vi "Visible Label.vi"(8 "error in (no error)":errorcluster, 10 "label":enum8{"hide", "show"}(ring), 11 "GObject in":refnum<vi>) -> (0 "error out":errorcluster, 1 "was label visible?":enum8{"hide", "show"}(ring), 2 "has label?":bool, 3 "GObject out":refnum<vi>)   [LabVIEW 2019, in "Builtins.lvlib"]
doc: "Shows or hides the GObject label if exists.\n\nCreated by: Ryan Pacini"
uses:
  Builtins.lvlib
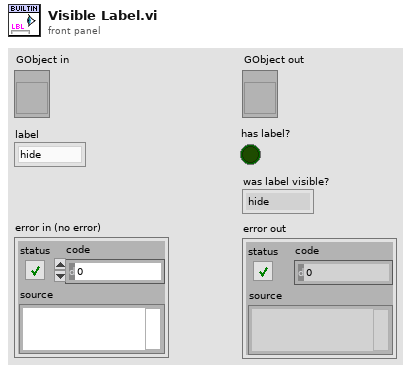
[diagram p1: front panel]
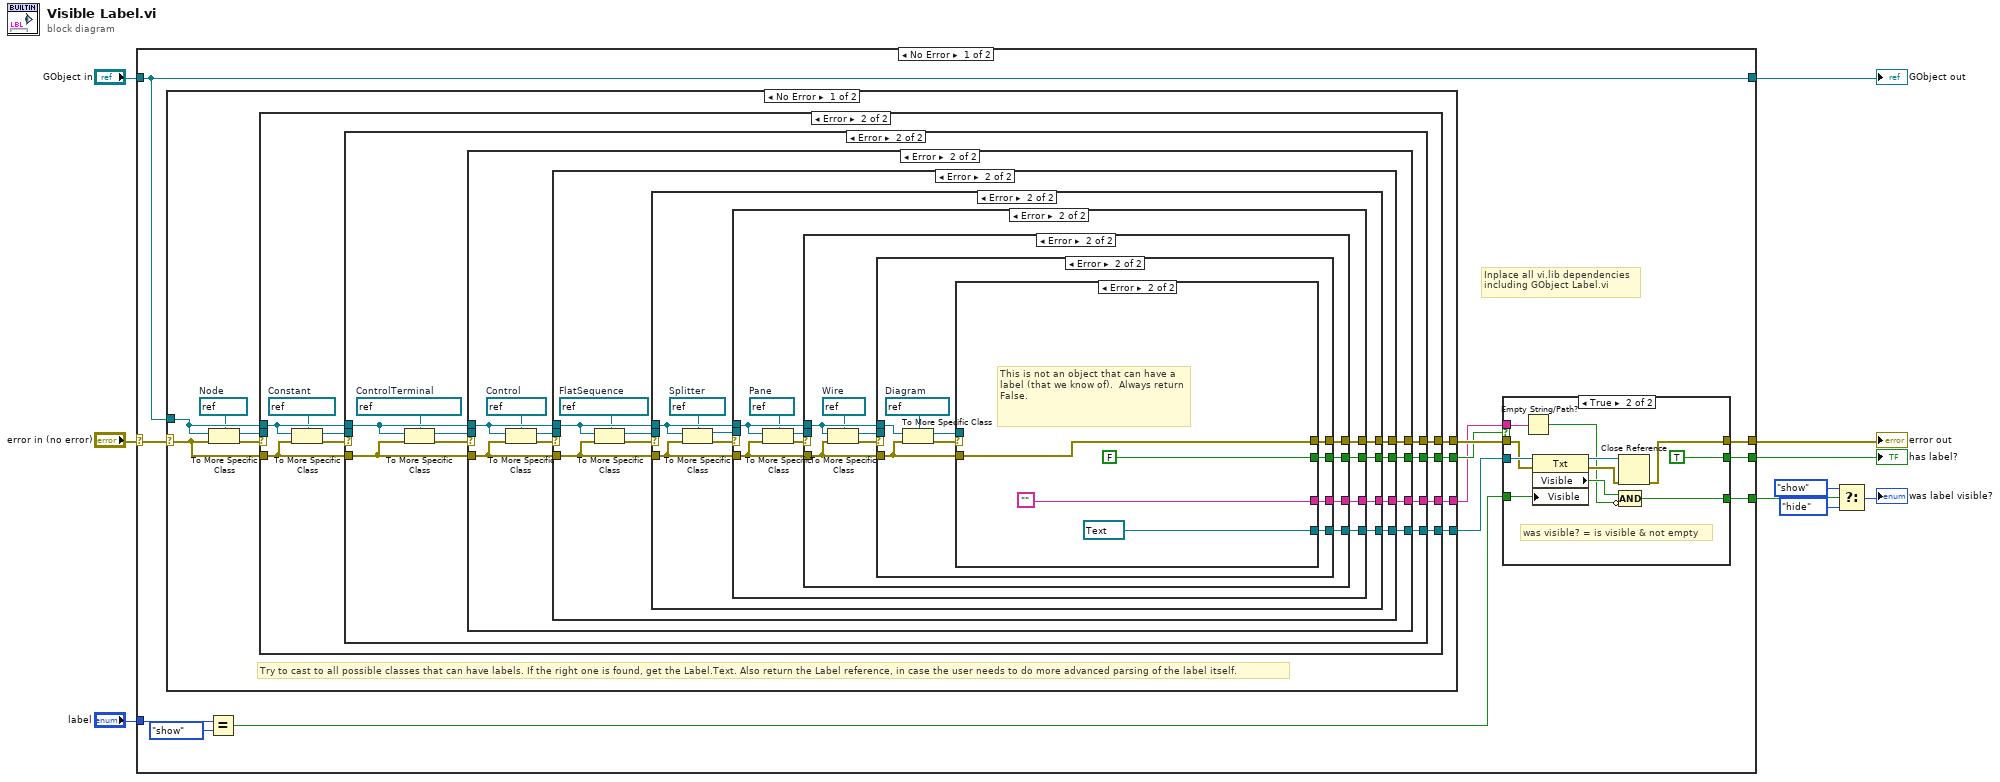
[diagram p0: block diagram]
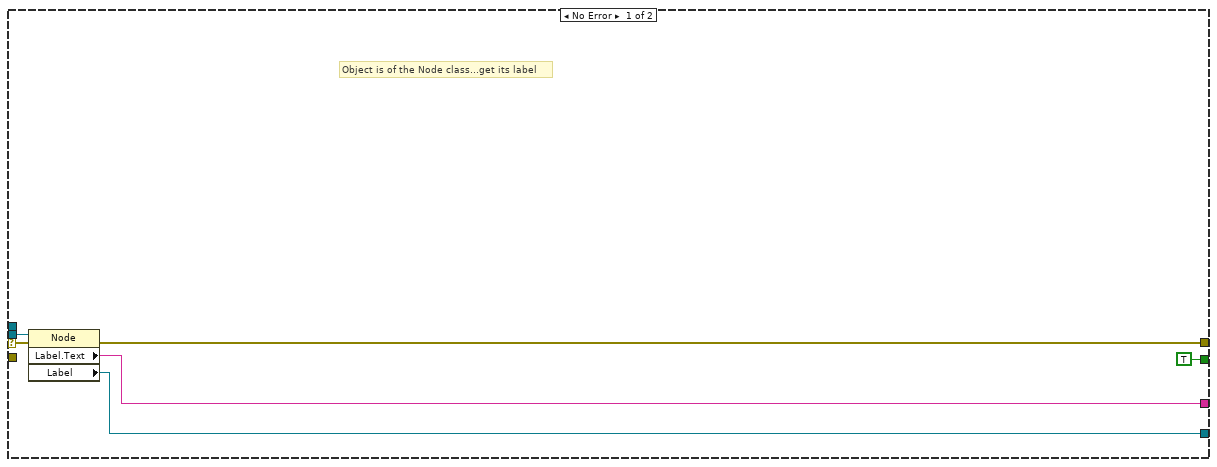
[diagram p2: hidden frame]
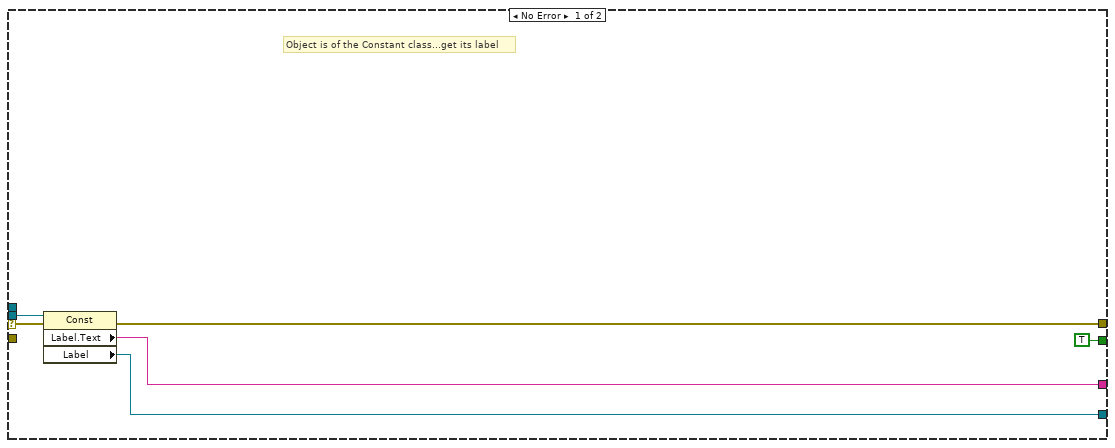
[diagram p3: hidden frame]
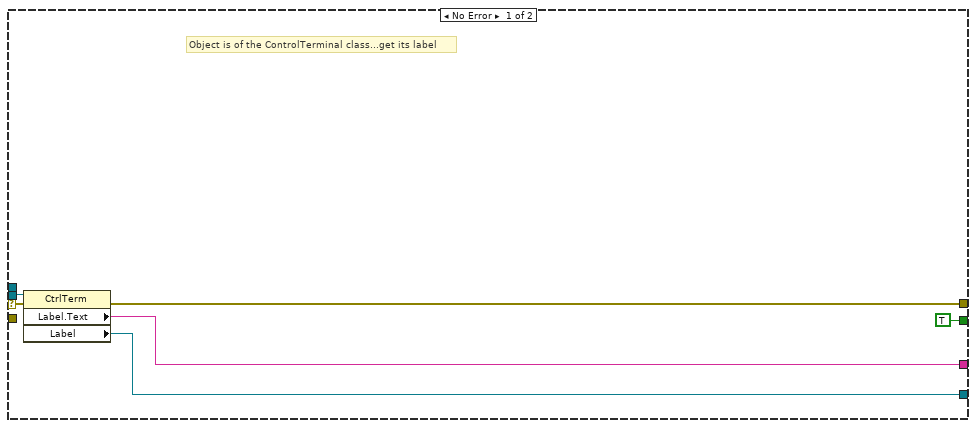
[diagram p4: hidden frame]
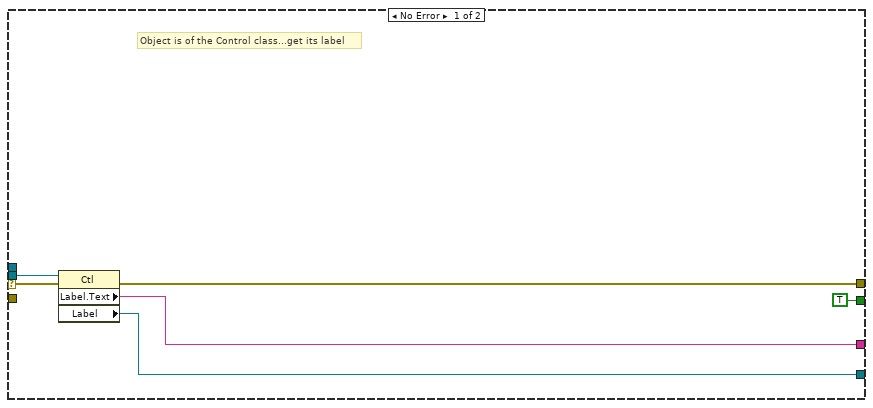
[diagram p5: hidden frame]
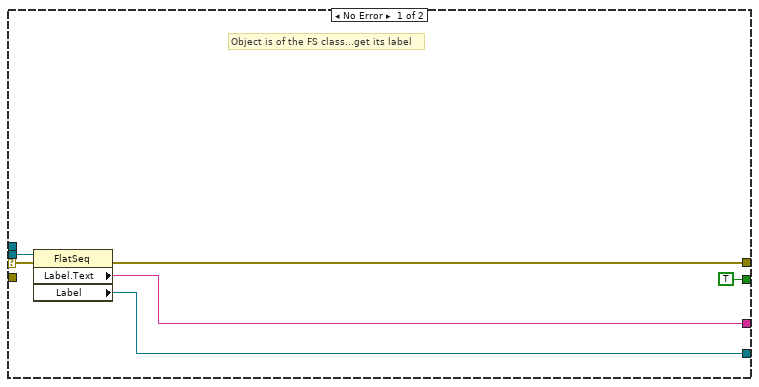
[diagram p6: hidden frame]
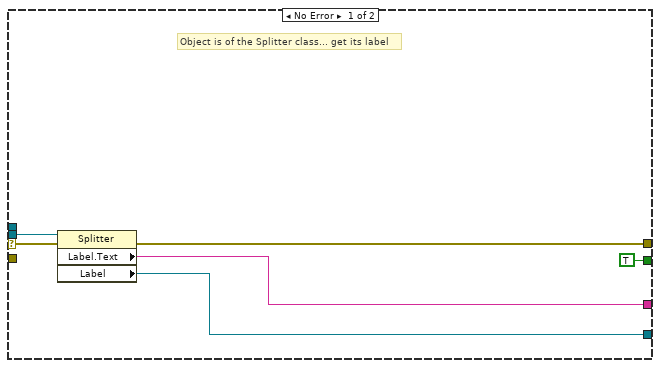
[diagram p7: hidden frame]
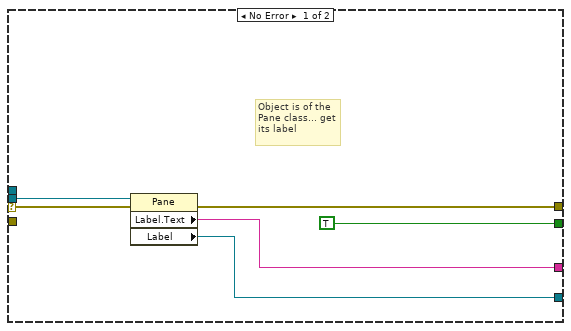
[diagram p8: hidden frame]
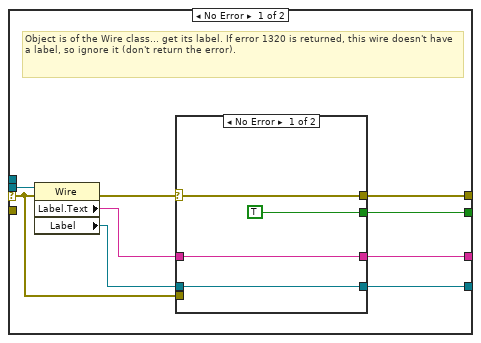
[diagram p9: hidden frame]
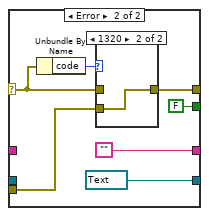
[diagram p10: hidden frame]
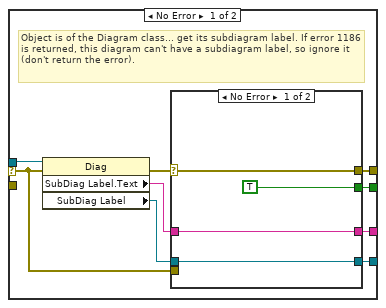
[diagram p12: hidden frame]
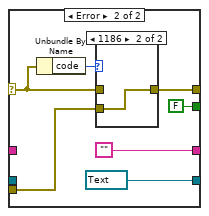
[diagram p13: hidden frame]
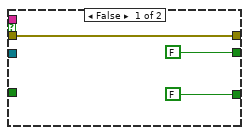
[diagram p16: hidden frame]
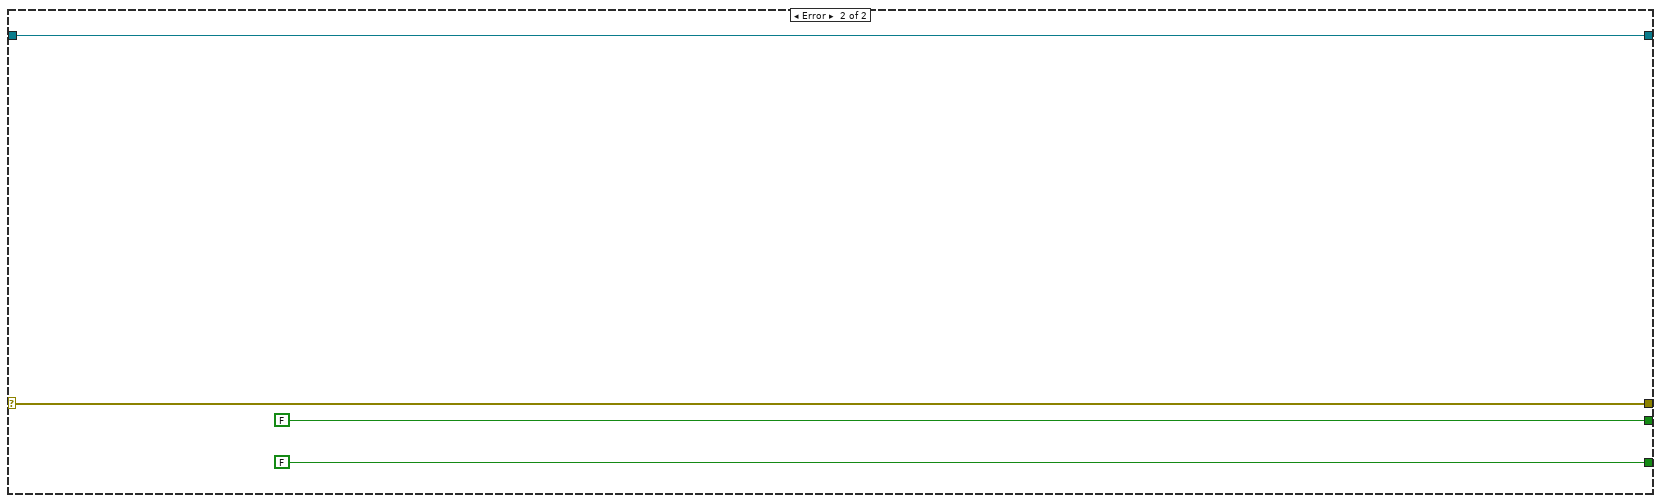
[diagram p17: hidden frame]
diagram:
  n1 = case shown="No Error" "error in (no error)" {
    selector: "error in (no error)" -> [w22 w211]
    tunnel: "label" -> [w14 _]
    tunnel: [w19 FALSE ("Visible")] -> w5
    tunnel: [w18 w211] -> w4
    tunnel: "GObject in" -> [w16 w212]
    tunnel: [w16 w212] -> w2
    tunnel: [w15 FALSE] -> w1
    frame No Error {
      # "Inplace all vi.lib dependencies\nincluding GObject Label.vi"
      n2 = case shown="No Error" w22 {
        selector: w22 -> [w27 w194]
        tunnel: w16 -> [w26 _]
        tunnel: [w31 w194] -> w20
        tunnel: [w30 _] -> w17
        tunnel: [w25 _] -> w11
        tunnel: [w24 _] -> w21
        frame No Error {
          w23 = refnum<vi> refnum  # Node
          # "Try to cast to all possible classes that can have labels. If the right one is found, get the Label.Text. Also return the Label reference, in case the user needs to do more advanced parsing of the label itself."
          n3 = To More Specific Class(target class=w23, reference=w26, error in=w27) -> (specific class reference=w28:refnum<vi>, error out=w29:errorcluster)
          n4 = case shown="Error" w29 {
            selector: w29 -> [w37 _]
            tunnel: w26 -> [_ w44]
            tunnel: w28 -> [w36 _]
            tunnel: w27 -> [_ w43]
            tunnel: [TRUE w42] -> w30
            tunnel: [w35 w41] -> w31
            tunnel: [w33 w40] -> w25
            tunnel: [w32 w39] -> w24
            frame No Error {
              # "Object is of the Node class...get its label"
              n5 = property class="Node"(reference=w36, error in=w37) -> (error out=w35:errorcluster, "Label.Text"=w33:string, "Label"=w32:refnum<vi>)  [unwired: 1 out]
            }
            frame Error {
              w38 = refnum<vi> refnum  # Constant
              n6 = To More Specific Class(target class=w38, reference=w44, error in=w43) -> (specific class reference=w45:refnum<vi>, error out=w46:errorcluster)
              n7 = case shown="Error" w46 {
                selector: w46 -> [w52 _]
                tunnel: w45 -> [w51 _]
                tunnel: w44 -> [_ w59]
                tunnel: w43 -> [_ w58]
                tunnel: [TRUE w56] -> w42
                tunnel: [w50 w57] -> w41
                tunnel: [w48 w55] -> w40
                tunnel: [w47 w54] -> w39
                frame No Error {
                  # "Object is of the Constant class...get its label"
                  n8 = property class="Const"(reference=w51, error in=w52) -> (error out=w50:errorcluster, "Label.Text"=w48:string, "Label"=w47:refnum<vi>)  [unwired: 1 out]
                }
                frame Error {
                  w53 = refnum<vi> refnum  # ControlTerminal
                  n9 = To More Specific Class(target class=w53, reference=w59, error in=w58) -> (specific class reference=w60:refnum<vi>, error out=w61:errorcluster)
                  n10 = case shown="Error" w61 {
                    selector: w61 -> [w67 _]
                    tunnel: w60 -> [w66 _]
                    tunnel: w59 -> [_ w74]
                    tunnel: w58 -> [_ w73]
                    tunnel: [w65 w72] -> w57
                    tunnel: [TRUE w71] -> w56
                    tunnel: [w64 w70] -> w55
                    tunnel: [w62 w69] -> w54
                    frame No Error {
                      # "Object is of the ControlTerminal class...get its label"
                      n11 = property class="CtrlTerm"(reference=w66, error in=w67) -> (error out=w65:errorcluster, "Label.Text"=w64:string, "Label"=w62:refnum<vi>)  [unwired: 1 out]
                    }
                    frame Error {
                      w68 = refnum<vi> refnum  # Control
                      n12 = To More Specific Class(target class=w68, reference=w74, error in=w73) -> (specific class reference=w75:refnum<vi>, error out=w76:errorcluster)
                      n13 = case shown="Error" w76 {
                        selector: w76 -> [w82 _]
                        tunnel: w75 -> [w81 _]
                        tunnel: w74 -> [_ w86]
                        tunnel: w73 -> [_ w89]
                        tunnel: [w80 w87] -> w72
                        tunnel: [TRUE w88] -> w71
                        tunnel: [w79 w85] -> w70
                        tunnel: [w77 w84] -> w69
                        frame No Error {
                          # "Object is of the Control class...get its label"
                          n14 = property class="Ctl"(reference=w81, error in=w82) -> (error out=w80:errorcluster, "Label.Text"=w79:string, "Label"=w77:refnum<vi>)  [unwired: 1 out]
                        }
                        frame Error {
                          w83 = refnum<vi> refnum  # FlatSequence
                          n15 = To More Specific Class(target class=w83, reference=w86, error in=w89) -> (specific class reference=w90:refnum<vi>, error out=w91:errorcluster)
                          n16 = case shown="Error" w91 {
                            selector: w91 -> [w97 _]
                            tunnel: w90 -> [w96 _]
                            tunnel: w89 -> [_ w104]
                            tunnel: [TRUE w101] -> w88
                            tunnel: [w95 w102] -> w87
                            tunnel: w86 -> [_ w105]
                            tunnel: [w94 w100] -> w85
                            tunnel: [w92 w99] -> w84
                            frame No Error {
                              # "Object is of the FS class...get its label"
                              n17 = property class="FlatSeq"(reference=w96, error in=w97) -> (error out=w95:errorcluster, "Label.Text"=w94:string, "Label"=w92:refnum<vi>)  [unwired: 1 out]
                            }
                            frame Error {
                              w98 = refnum<vi> refnum  # Splitter
                              n18 = To More Specific Class(target class=w98, reference=w105, error in=w104) -> (specific class reference=w103:refnum<vi>, error out=w106:errorcluster)
                              n19 = case shown="Error" w106 {
                                selector: w106 -> [w110 _]
                                tunnel: w105 -> [_ w115]
                                tunnel: w104 -> [_ w120]
                                tunnel: w103 -> [w112 _]
                                tunnel: [w111 w119] -> w102
                                tunnel: [TRUE w118] -> w101
                                tunnel: [w109 w116] -> w100
                                tunnel: [w107 w114] -> w99
                                frame No Error {
                                # "Object is of the Splitter class... get its label"
                                n20 = property class="Splitter"(reference=w112, error in=w110) -> (error out=w111:errorcluster, "Label.Text"=w109:string, "Label"=w107:refnum<vi>)  [unwired: 1 out]
                                }
                                frame Error {
                                w113 = refnum<vi> refnum  # Pane
                                n21 = To More Specific Class(target class=w113, reference=w115, error in=w120) -> (specific class reference=w117:refnum<vi>, error out=w121:errorcluster)
                                n22 = case shown="Error" w121 {
                                selector: w121 -> [w127 _]
                                tunnel: w120 -> [_ w132]
                                tunnel: [w125 w131] -> w119
                                tunnel: [TRUE w136] -> w118
                                tunnel: w117 -> [w126 _]
                                tunnel: [w124 w135] -> w116
                                tunnel: w115 -> [_ w130]
                                tunnel: [w122 w129] -> w114
                                frame No Error {
                                # "Object is of the Pane class... get its label"
                                n23 = property class="Pane"(reference=w126, error in=w127) -> (error out=w125:errorcluster, "Label.Text"=w124:string, "Label"=w122:refnum<vi>)  [unwired: 1 out]
                                }
                                frame Error {
                                w128 = refnum<vi> refnum  # Wire
                                n24 = To More Specific Class(target class=w128, reference=w130, error in=w132) -> (specific class reference=w133:refnum<vi>, error out=w134:errorcluster)
                                n25 = case shown="Error" w134 {
                                selector: w134 -> [w141 _]
                                tunnel: [w139 w167] -> w136
                                tunnel: [w138 w166] -> w135
                                tunnel: w133 -> [w145 _]
                                tunnel: w132 -> [_ w162]
                                tunnel: [w140 w161] -> w131
                                tunnel: w130 -> [_ w165]
                                tunnel: [w137 w160] -> w129
                                frame No Error {
                                # "Object is of the Wire class... get its label. If error 1320 is returned, this wire doesn't have a label, so ignore it (don't return the error)."
                                n26 = property class="Wire"(reference=w145, error in=w141) -> (error out=w144:errorcluster, "Label.Text"=w143:string, "Label"=w142:refnum<vi>)  [unwired: 1 out]
                                n27 = case shown="No Error" w144 {
                                selector: w144 -> [w149 w155]
                                tunnel: [w149 w152] -> w140
                                tunnel: w143 -> [w148 _]
                                tunnel: [w148 ""] -> w138
                                tunnel: w142 -> [w146 _]
                                tunnel: [w146 refnum<vi> refnum ("SubDiag Label")] -> w137
                                tunnel: [TRUE FALSE] -> w139
                                tunnel: w141 -> [_ w150]
                                frame No Error {
                                }
                                frame Error {
                                n28 = Unbundle By Name(w155) -> ("code"=w156:i32)
                                n29 = case shown="1320" w156 {
                                tunnel: w155 -> [w157 _]
                                tunnel: [w157 w158] -> w152
                                tunnel: w150 -> [_ w158]
                                frame Default {
                                }
                                frame 1320 {
                                }
                                }
                                }
                                }
                                }
                                frame Error {
                                w159 = refnum<vi> refnum  # Diagram
                                n30 = To More Specific Class(target class=w159, reference=w165, error in=w162) -> (specific class reference=w163:refnum<vi>, error out=w164:errorcluster)
                                n31 = case shown="Error" w164 {
                                selector: w164 -> [w168 _]
                                tunnel: [w169 FALSE] -> w167
                                tunnel: [w173 ""] -> w166
                                tunnel: w163 -> [w176 _]
                                tunnel: w162 -> [_ w191]
                                tunnel: [w174 w191] -> w161
                                tunnel: [w171 refnum<vi> refnum ("SubDiag Label")] -> w160
                                frame No Error {
                                # "Object is of the Diagram class... get its subdiagram label. If error 1186 is returned, this diagram can't have a subdiagram label, so ignore it (don't return the error)."
                                n32 = property class="Diag"(reference=w176, error in=w168) -> (error out=w175:errorcluster, "SubDiag Label.Text"=w172:string, "SubDiag Label"=w170:refnum<vi>)  [unwired: 1 out]
                                n33 = case shown="No Error" w175 {
                                selector: w175 -> [w180 w186]
                                tunnel: [w180 w183] -> w174
                                tunnel: w172 -> [w179 _]
                                tunnel: [w179 ""] -> w173
                                tunnel: w170 -> [w177 _]
                                tunnel: [w177 refnum<vi> refnum ("SubDiag Label")] -> w171
                                tunnel: [TRUE FALSE] -> w169
                                tunnel: w168 -> [_ w181]
                                frame No Error {
                                }
                                frame Error {
                                n34 = Unbundle By Name(w186) -> ("code"=w187:i32)
                                n35 = case shown="1186" w187 {
                                tunnel: w186 -> [w188 _]
                                tunnel: [w188 w189] -> w183
                                tunnel: w181 -> [_ w189]
                                frame Default {
                                }
                                frame 1186 {
                                }
                                }
                                }
                                }
                                }
                                frame Error {
                                # "This is not an object that can have a label (that we know of).  Always return False."
                                }
                                }
                                }
                                }
                                }
                                }
                                }
                              }
                            }
                          }
                        }
                      }
                    }
                  }
                }
              }
            }
          }
        }
        frame Error {
        }
      }
      n36 = Equal?(x=w14, y=enum8{"hide", "show"}."show") -> (x = y?=w13:bool)
      n37 = case shown="True" w17 {
        tunnel: w21 -> [_ w208]
        tunnel: w20 -> [w197 w207]
        tunnel: w13 -> [_ w206]
        tunnel: [FALSE ("Visible") w199] -> w19
        tunnel: [w197 w203] -> w18
        tunnel: [FALSE TRUE] -> w15
        tunnel: w11 -> [_ w201]
        frame False {
        }
        frame True {
          # "was visible? = is visible & not empty"
          n38 = Empty String/Path?(string/path=w201) -> (empty?=w198:bool)
          n39 = property class="Txt"(reference=w208, error in=w207, "Visible"=w206) -> (reference out=w205:refnum<vi>, error out=w204:errorcluster, "Visible"=w200:bool)
          n40 = Close Reference(reference=w205, error in (no error)=w204) -> (error out=w203:errorcluster)
          n41 = Compound Arithmetic op=AND(w200, invert w198) -> (w199:bool)
        }
      }
    }
    frame Error {
    }
  }
  "error out" <- w4
  "GObject out" <- w2
  "has label?" <- w1
  n42 = Select(t=enum8{"hide", "show"}."show" ("was inc/dec visible?"), s=w5, f=enum8{"hide", "show"}."hide" ("was inc/dec visible?")) -> (s? t:f=→"was label visible?":enum8{"hide", "show"})
